vi "string2double.vi"(1 "String":string="1ns") -> (0 "double":dbl)   [LabVIEW 2021]
doc: "This VI converts an SI unit string to double. (1ns, 1k, 1mA, 100Hz, etc.)\nIt will remove the last character from the string if it is an unknown unit / prefix.\nFor frequency parameters it will remove the last tw characters.\nAlso works with regular numbers (100, 0.001, 1E-6).\nWhen a String contains the characters \"0x\" it is detected as hexadecimal and converted accordingly"
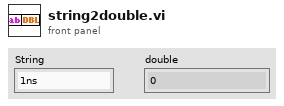
[diagram p1: front panel]
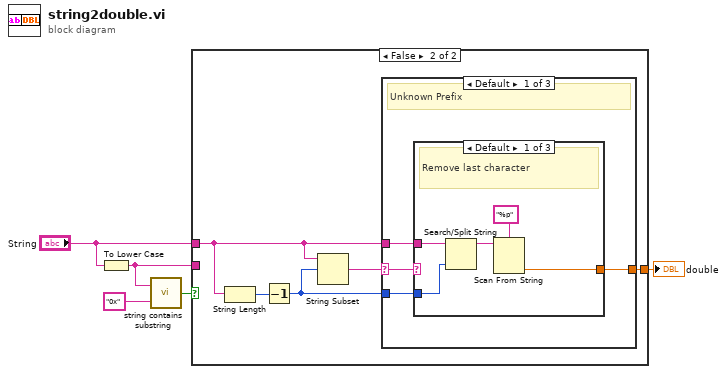
[diagram p0: block diagram]
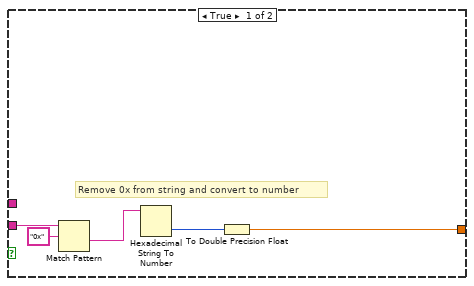
[diagram p2: hidden frame]
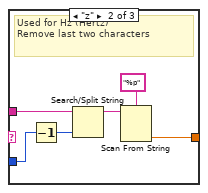
[diagram p3: hidden frame]
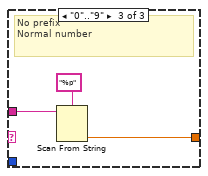
[diagram p4: hidden frame]
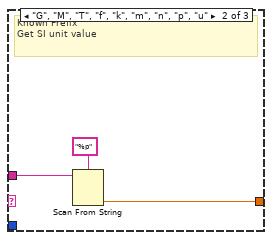
[diagram p5: hidden frame]
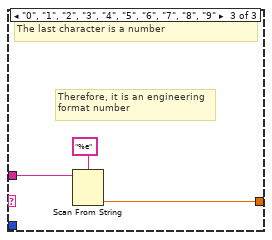
[diagram p6: hidden frame]
diagram:
  n1 = To Lower Case(string="String") -> (all lower case string=w1:string)
  n2 = call "string contains substring.vi"("Search String"="0x", "Input String"=w1) -> ("Found?"=w3:bool)
  n3 = case shown="False" w3 {
    tunnel: "String" -> [_ w15]
    tunnel: [w9 w12] -> w4
    tunnel: w1 -> [w8 _]
    frame True {
      # "Remove 0x from string and convert to number"
      n4 = Match Pattern(string=w8, regular expression="0x") -> (after substring=w6:string)  [unwired: 1 in, 3 out]
      n5 = Hexadecimal String To Number(string=w6) -> (number=w10:u32)  [unwired: 2 in, 1 out]
      n6 = To Double Precision Float(number=w10) -> (double precision float=w9:dbl)
    }
    frame False {
      n7 = String Length(string=w15) -> (length=w14:i32)
      n8 = Decrement(x=w14) -> (x-1=w11:i32)
      n9 = String Subset(string=w15, offset (0)=w11) -> (substring=w13:string)  [unwired: 1 in]
      n10 = case shown="Default" w13 {
        selector: w13 -> [w19 _ _]
        tunnel: w15 -> [w18 w35 w38]
        tunnel: [w17 w34 w37] -> w12
        tunnel: w11 -> [w16 _ _]
        frame Default {
          # "Unknown Prefix"
          n11 = case shown="Default" w19 {
            tunnel: w18 -> [w24 w30 w32]
            tunnel: [w20 w27 w31] -> w17
            tunnel: w16 -> [w23 w26 _]
            frame Default {
              # "Remove last character"
              n12 = Search/Split String(string=w24, offset (0)=w23) -> (substring before match=w21:string)  [unwired: 1 in, 2 out]
              n13 = Scan From String(format string="%p", input string=w21) -> (output 1=w20:dbl)  [unwired: 3 in, 3 out]
            }
            frame "z" {
              # "Used for Hz (Hertz)\nRemove last two characters"
              n14 = Decrement(x=w26) -> (x-1=w25:i32)
              n15 = Search/Split String(string=w30, offset (0)=w25) -> (substring before match=w28:string)  [unwired: 1 in, 2 out]
              n16 = Scan From String(format string="%p", input string=w28) -> (output 1=w27:dbl)  [unwired: 3 in, 3 out]
            }
            frame "0".."9" {
              # "No prefix\nNormal number"
              n17 = Scan From String(format string="%p", input string=w32) -> (output 1=w31:dbl)  [unwired: 3 in, 3 out]
            }
          }
        }
        frame "G", "M", "T", "f", "k", "m", "n", "p", "u" {
          # "Known Prefix\nGet SI unit value"
          n18 = Scan From String(format string="%p", input string=w35) -> (output 1=w34:dbl)  [unwired: 3 in, 3 out]
        }
        frame "0", "1", "2", "3", "4", "5", "6", "7", "8", "9" {
          # "Therefore, it is an engineering\nformat number"
          # "The last character is a number"
          n19 = Scan From String(format string="%e", input string=w38) -> (output 1=w37:dbl)  [unwired: 3 in, 3 out]
        }
      }
    }
  }
  "double" <- w4
